vi "隐藏页面.vi"() -> ()   [LabVIEW 2019]
panel:
  in  "停止":bool
  out "数值":i32
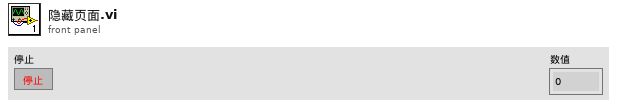
[diagram p1: front panel]
types:
  T1 = enum16{"Always On", "Always Off", "Off While Running"}
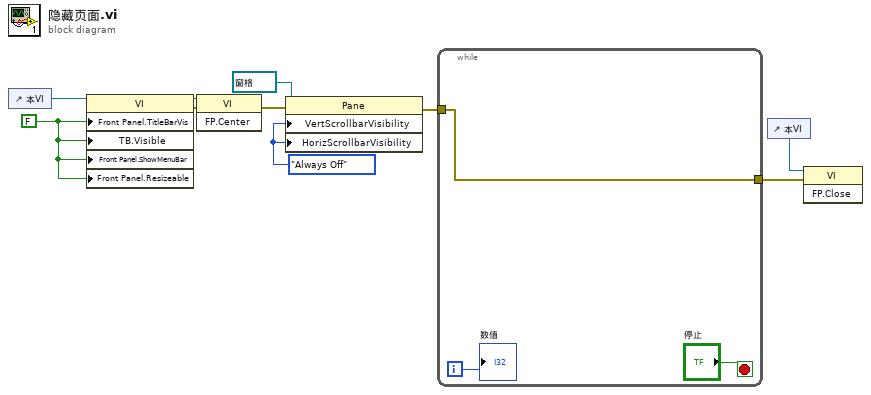
[diagram p0: block diagram]
diagram:
  w10 = T1."Always Off" ("垂直滚动条可见")
  w9 = FALSE ("前面板窗口:标题栏可见")
  n1 = control-ref of="本VI"() -> (w8:refnum<vi>)
  n2 = property class="VI"(reference=w8, "Front Panel.TitleBarVis"=w9, "TB.Visible"=w9, "Front Panel.ShowMenuBar"=w9, "Front Panel.Resizeable"=w9) -> (reference out=w7:refnum<vi>, error out=w6:errorcluster)  [unwired: 1 in]
  n3 = invoke class="VI" method="FP.Center"(reference=w7, error in=w6) -> (error out=w5:errorcluster)  [unwired: 1 in, 2 out]
  n4 = property class="Pane"(reference=refnum<vi> refnum ("引用"), error in=w5, "VertScrollbarVisibility"=w10, "HorizScrollbarVisibility"=w10) -> (error out=w3:errorcluster)  [unwired: 1 out]
  n5 = while {
    tunnel: w3 -> [w11]
    tunnel: [w11] -> w2
    i -> [w13]
    stop <- "停止" stop-if-true
    "数值" <- w13
  }
  n6 = control-ref of="本VI"() -> (w4:refnum<vi>)
  n7 = invoke class="VI" method="FP.Close"(reference=w4, error in=w2) -> ()  [unwired: 1 in, 3 out]
